vi "Vision Auto Target_Old.vi"(11 "navX Device":T1={"Interface"={"Protocol"=enum."SERIAL", "Update Rate (4Hz-60Hz)"=4, "navX Open TypeDef"=variant}, "Notify Packet"=refnum, "Loop VI Refnum"=refnum, "Ready to Close Occurrence Refnum"=refnum} {"Interface"."Update Rate (4Hz-60Hz)" min=4 max=60 step=1}) -> ()   [LabVIEW 2015]
uses:
  NavX/navX Library v2/TypeDefs/Z900_navX_DeviceTypeDef.ctl
  NavX/navX Library v2/TypeDefs/Z900_navX_ProtocolTypeDef.ctl
  NavX/navX Library v2/TypeDefs/Z900_navX_NotifyPacketTypeDef.ctl
  NavX/navX Library v2/TypeDefs/Z900_navX_ActionTypeDef.ctl
  Team Code/Robot Global Data.vi
  <vilib>/Rock Robotics/Network Tables/NT Write Number.vi
  NavX/navX Library v2/navX Library v2.lvlib
panel:
  in  "Y Gain":dbl=6.5
  in  "Y at Defenses":dbl=-0.4
  in  "InvGain":dbl=80.0
  in  "minimumVisionValue":dbl=0.45
  out "Waveform Chart":cluster{"VisionGyroTarget":dbl, dbl, dbl}(graph)
  out "VisionState":enum16{"Disabled", "Enable", "Suspended", "PID"}(ring)
  in  "Offset":dbl=0.05
  # "0.05 = 4 inches from defenses\n- = Left\n+ = Right"
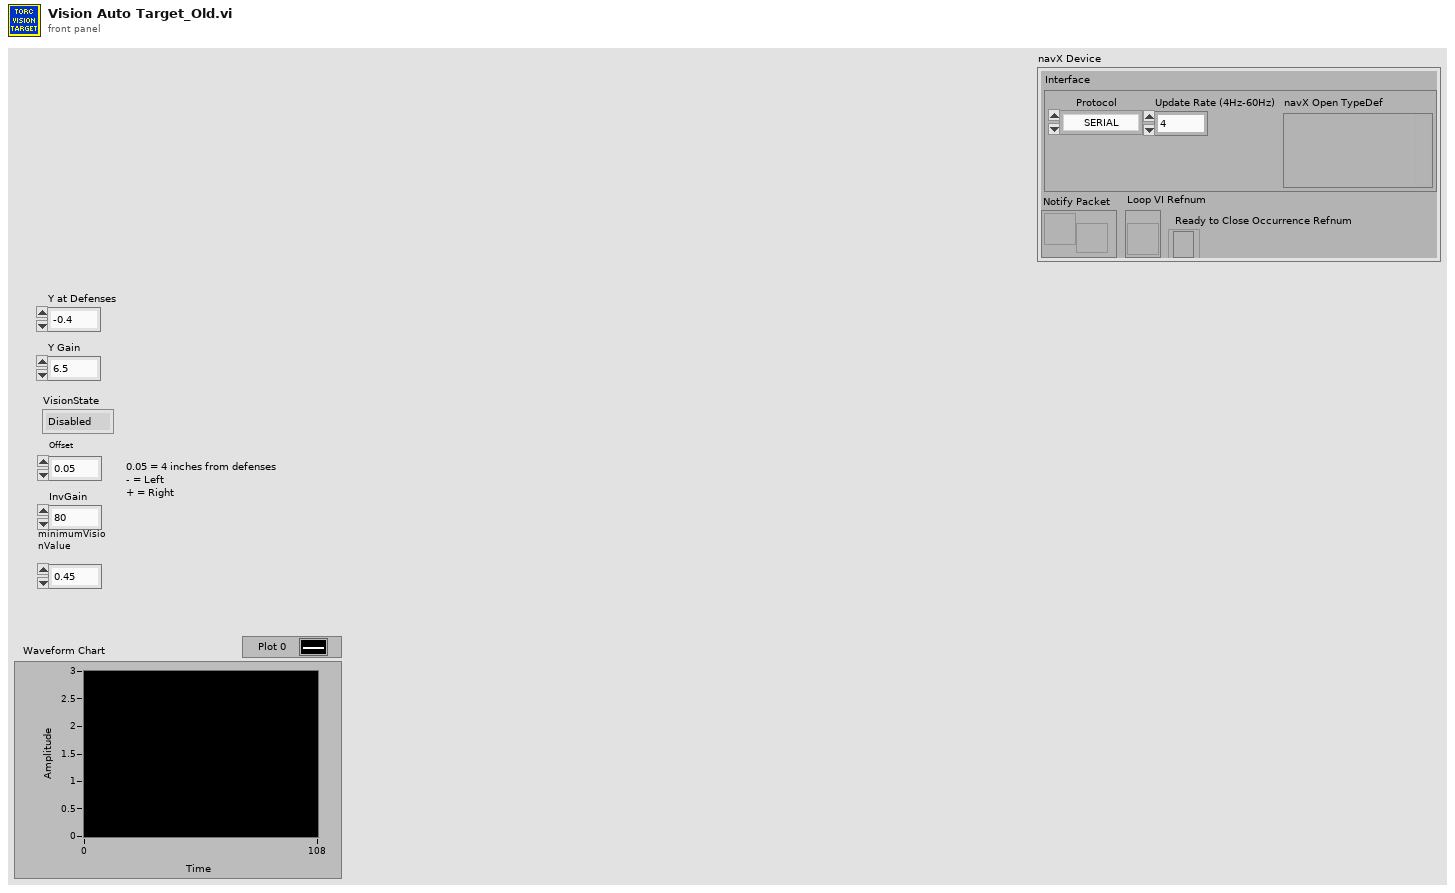
[diagram p1: front panel]
types:
  T1 = typedef "navX Library v2.lvlib/Z900_navX_DeviceTypeDef.ctl" = cluster{"Interface":cluster{"Protocol":T2, "Update Rate (4Hz-60Hz)":u8, "navX Open TypeDef":variant}, "Notify Packet":refnum<notifier>, "Loop VI Refnum":refnum<vi>, "Ready to Close Occurrence Refnum":refnum<k4>}
  T2 = typedef "navX Library v2.lvlib/Z900_navX_ProtocolTypeDef.ctl" = enum16{"SERIAL", "I2C", "SPI"}
  T3 = cluster{"Yaw":dbl, "Roll":dbl, "Pitch":dbl, "Heading":dbl, "Fused Heading":dbl}
  T4 = cluster{"Distance (ft)":dbl, "Center":cluster{dbl, dbl}, "Normalized Rect":cluster{"Numeric":dbl, "Numeric 2":dbl, "Numeric 3":dbl, "Numeric 5":dbl}}[]
  T5 = cluster{"Detected Targets[0]":cluster{"Distance (ft)":dbl, "Center":cluster{dbl, dbl}, "Normalized Rect":cluster{"Numeric":dbl, "Numeric 2":dbl, "Numeric 3":dbl, "Numeric 5":dbl}}, "Detected Targets[1]":cluster{"Distance (ft)":dbl, "Center":cluster{dbl, dbl}, "Normalized Rect":cluster{"Numeric":dbl, "Numeric 2":dbl, "Numeric 3":dbl, "Numeric 5":dbl}}, "Detected Targets[2]":cluster{"Distance (ft)":dbl, "Center":cluster{dbl, dbl}, "Normalized Rect":cluster{"Numeric":dbl, "Numeric 2":dbl, "Numeric 3":dbl, "Numeric 5":dbl}}, "Detected Targets[3]":cluster{"Distance (ft)":dbl, "Center":cluster{dbl, dbl}, "Normalized Rect":cluster{"Numeric":dbl, "Numeric 2":dbl, "Numeric 3":dbl, "Numeric 5":dbl}}, "Detected Targets[4]":cluster{"Distance (ft)":dbl, "Center":cluster{dbl, dbl}, "Normalized Rect":cluster{"Numeric":dbl, "Numeric 2":dbl, "Numeric 3":dbl, "Numeric 5":dbl}}, "Detected Targets[5]":cluster{"Distance (ft)":dbl, "Center":cluster{dbl, dbl}, "Normalized Rect":cluster{"Numeric":dbl, "Numeric 2":dbl, "Numeric 3":dbl, "Numeric 5":dbl}}, "Detected Targets[6]":cluster{"Distance (ft)":dbl, "Center":cluster{dbl, dbl}, "Normalized Rect":cluster{"Numeric":dbl, "Numeric 2":dbl, "Numeric 3":dbl, "Numeric 5":dbl}}, "Detected Targets[7]":cluster{"Distance (ft)":dbl, "Center":cluster{dbl, dbl}, "Normalized Rect":cluster{"Numeric":dbl, "Numeric 2":dbl, "Numeric 3":dbl, "Numeric 5":dbl}}, "Detected Targets[8]":cluster{"Distance (ft)":dbl, "Center":cluster{dbl, dbl}, "Normalized Rect":cluster{"Numeric":dbl, "Numeric 2":dbl, "Numeric 3":dbl, "Numeric 5":dbl}}}
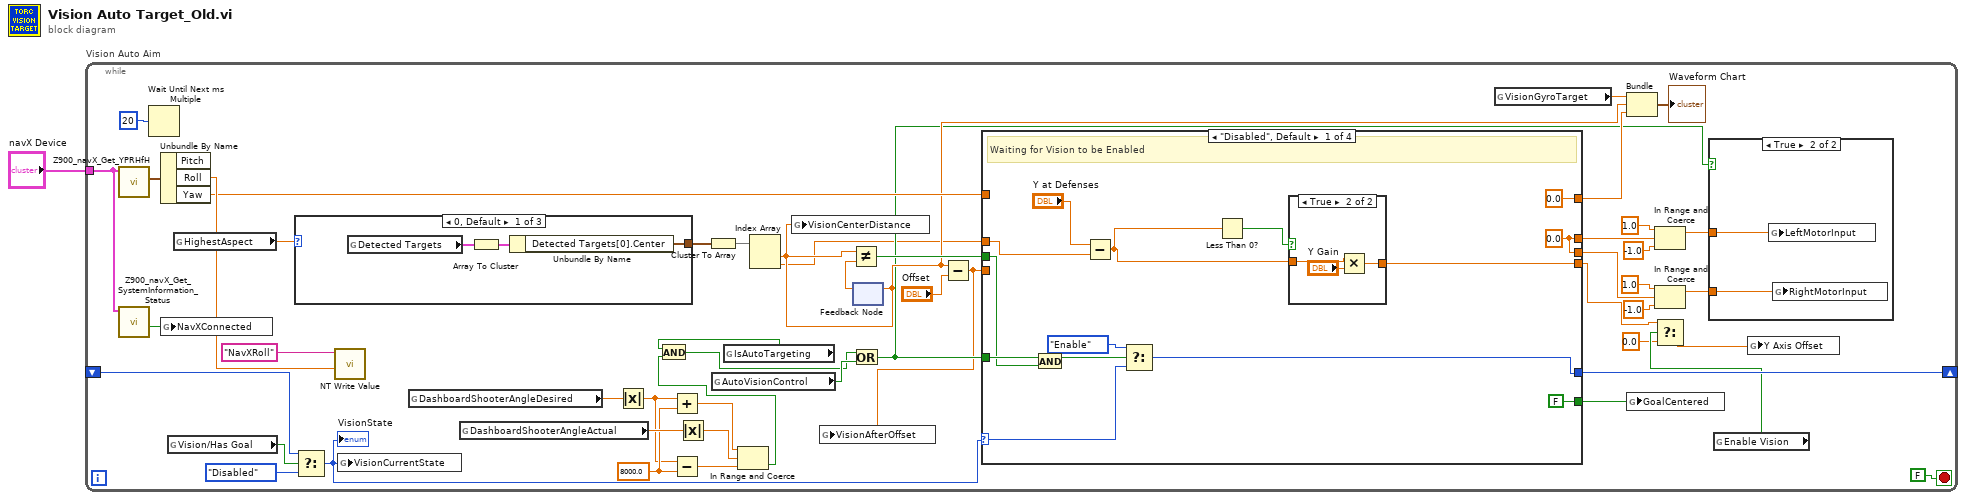
[diagram p0: block diagram]
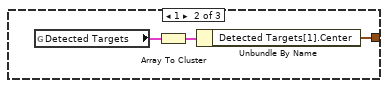
[diagram p2: hidden frame]
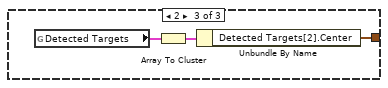
[diagram p3: hidden frame]
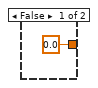
[diagram p5: hidden frame]
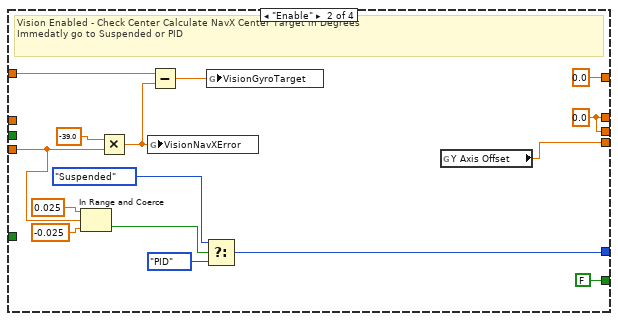
[diagram p6: hidden frame]
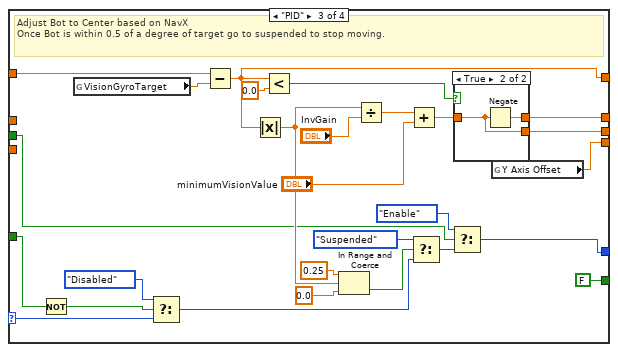
[diagram p7: hidden frame]
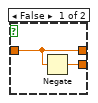
[diagram p8: hidden frame]
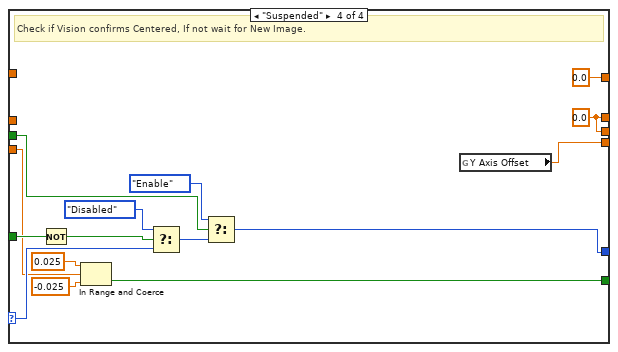
[diagram p9: hidden frame]
diagram:
  n1 = while "Vision Auto Aim" {
    tunnel: "navX Device" -> [w45]
    shift-right: [w48] -> _
    shift-left: _ -> [w26]
    stop <- FALSE stop-if-true
    w12 = 8000.0 ("y")
    n2 = call "Z900_navX_Get_YPRHfH.vi"("navX Device"=w45) -> ("YRPHfH"=w49:T3)  [unwired: 7 in, 3 out]
    n3 = call "Z900_navX_Get_SystemInformation_Status.vi"("navX Device"=w45) -> ("Connected"=w28:bool)  [unwired: 7 in, 3 out]
    n4 = Wait Until Next ms Multiple(millisecond multiple=u32 20 ("milliseconds to wait")) -> ()  [unwired: 1 out]
    n5 = Unbundle By Name(w49) -> ("Roll"=w47:dbl, "Yaw"=w21:dbl)  [unwired: 1 out]
    n6 = global write "Robot Global Data.vi" "NavXConnected"(w28) -> ()
    n7 = global read "Robot Global Data.vi" "Vision/Has Goal"() -> (w25:bool)
    n8 = global read "Robot Global Data.vi" "HighestAspect"() -> (w23:dbl)
    n9 = case shown="0, Default" w23 {
      tunnel: [w52 w55 w58] -> w32
      frame 0, Default {
        n10 = global read "Robot Global Data.vi" "Detected Targets"() -> (w53:T4)
        n11 = Array To Cluster(array=w53) -> (cluster=w54:T5)
        n12 = Unbundle By Name(w54) -> ("Detected Targets[0].Center"=w52:cluster{dbl, dbl})
      }
      frame 1 {
        n13 = global read "Robot Global Data.vi" "Detected Targets"() -> (w56:T4)
        n14 = Array To Cluster(array=w56) -> (cluster=w57:T5)
        n15 = Unbundle By Name(w57) -> ("Detected Targets[1].Center"=w55:cluster{dbl, dbl})
      }
      frame 2 {
        n16 = global read "Robot Global Data.vi" "Detected Targets"() -> (w59:T4)
        n17 = Array To Cluster(array=w59) -> (cluster=w60:T5)
        n18 = Unbundle By Name(w60) -> ("Detected Targets[2].Center"=w58:cluster{dbl, dbl})
      }
    }
    n19 = Select(t=w26, s=w25, f=enum16{"Disabled", "Enable", "Suspended", "PID"}."Disabled" ("t")) -> (s? t:f=w27:enum16{"Disabled", "Enable", "Suspended", "PID"})
    "VisionState" <- w27
    n20 = call-poly <vilib>:"NT Write Value.vi"("Numeric"=w47, "Name"="NavXRoll") -> ()  [unwired: 9 in, 1 out]
    n21 = global write "Robot Global Data.vi" "VisionCurrentState"(w27) -> ()
    n22 = global read "Robot Global Data.vi" "DashboardShooterAngleDesired"() -> (w14:dbl)
    n23 = global read "Robot Global Data.vi" "DashboardShooterAngleActual"() -> (w17:dbl)
    n24 = Absolute Value(x=w14) -> (abs(x)=w11:dbl)
    n25 = Add(x=w11, y=w12) -> (x+y=w16:dbl)
    n26 = Subtract(x=w11, y=w12) -> (x-y=w15:dbl)
    n27 = Absolute Value(x=w17) -> (abs(x)=w13:dbl)
    n28 = Cluster To Array(cluster=w32) -> (array=w44:dbl[])
    n29 = global read "Robot Global Data.vi" "AutoVisionControl"() -> (w29:bool)
    n30 = global read "Robot Global Data.vi" "IsAutoTargeting"() -> (w10:bool)
    n31 = In Range and Coerce(upper limit=w16, x=w13, lower limit=w15) -> (In Range?=w9:bool)  [unwired: 1 out]
    n32 = And(x=w10, y=w9) -> (x .and. y?=w8:bool)
    n33 = Index Array(array=w44) -> (element #1=w20:dbl, element #2=w6:dbl)  [unwired: 2 in]
    n34 = global write "Robot Global Data.vi" "VisionCenterDistance"(w20) -> ()
    n35 = Or(x=w8, y=w29) -> (x .or. y?=w18:bool)
    n36 = feedback-in #1(w20) -> ()
    n37 = feedback #1() -> (w30:dbl)  [unwired: 1 in]
    n38 = Not Equal?(x=w20, y=w30) -> (x != y?=w31:bool)
    n39 = Subtract(x=w20, y="Offset") -> (x-y=w7:dbl)
    n40 = global write "Robot Global Data.vi" "VisionAfterOffset"(w7) -> ()
    n41 = case shown="\"Disabled\", Default" w27 {
      selector: w27 -> [w76 _ w99 w131]
      tunnel: w18 -> [w72 _ w102 w133]
      tunnel: [w74 w93 w104 w132] -> w48
      tunnel: w21 -> [_ w86 w111 _]
      tunnel: [FALSE FALSE FALSE w129] -> w19
      tunnel: w7 -> [_ w82 _ w128]
      tunnel: [w71 w89 w113 w141] -> w39
      tunnel: [w71 w89 w114 w141] -> w43
      tunnel: [0.0 0.0 w110 0.0] -> w34
      tunnel: w31 -> [w68 _ w98 w130]
      tunnel: w6 -> [w64 _ _ _]
      tunnel: [w65 w81 w97 w127] -> w4
      frame "Disabled", Default {
        w71 = 0.0
        # "Waiting for Vision to be Enabled"
        n42 = And(x=w72, y=w68) -> (x .and. y?=w69:bool)
        n43 = Subtract(x="Y at Defenses", y=w64) -> (x-y=w66:dbl)
        n44 = Select(t=enum16{"Disabled", "Enable", "Suspended", "PID"}."Enable", s=w69, f=w76) -> (s? t:f=w74:enum16{"Disabled", "Enable", "Suspended", "PID"})
        n45 = Less Than 0?(x=w66) -> (x < 0?=w67:bool)
        n46 = case shown="True" w67 {
          tunnel: w66 -> [_ w79]
          tunnel: [0.0 w78] -> w65
          frame False {
          }
          frame True {
            n47 = Multiply(x=w79, y="Y Gain") -> (x*y=w78:dbl)
          }
        }
      }
      frame "Enable" {
        w89 = 0.0 ("LeftMotorOutput")
        # "Vision Enabled - Check Center Calculate NavX Center Target in Degrees\nImmedatly go to Suspended or PID"
        n48 = In Range and Coerce(upper limit=0.025, x=w82, lower limit=-0.025) -> (In Range?=w84:bool)  [unwired: 1 out]
        n49 = Multiply(x=-39.0, y=w82) -> (x*y=w85:dbl)
        n50 = global write "Robot Global Data.vi" "VisionNavXError"(w85) -> ()
        n51 = Subtract(x=w86, y=w85) -> (x-y=w88:dbl)
        n52 = Select(t=enum16{"Disabled", "Enable", "Suspended", "PID"}."Suspended", s=w84, f=enum16{"Disabled", "Enable", "Suspended", "PID"}."PID" ("t")) -> (s? t:f=w93:enum16{"Disabled", "Enable", "Suspended", "PID"})
        n53 = global write "Robot Global Data.vi" "VisionGyroTarget"(w88) -> ()
        n54 = global read "Robot Global Data.vi" "Y Axis Offset"() -> (w81:dbl)
      }
      frame "PID" {
        # "Adjust Bot to Center based on NavX\nOnce Bot is within 0.5 of a degree of target go to suspended to stop moving."
        n55 = Not(x=w102) -> (.not. x?=w101:bool)
        n56 = global read "Robot Global Data.vi" "VisionGyroTarget"() -> (w120:dbl)
        n57 = Select(t=enum16{"Disabled", "Enable", "Suspended", "PID"}."Disabled", s=w101, f=w99) -> (s? t:f=w100:enum16{"Disabled", "Enable", "Suspended", "PID"})
        n58 = Subtract(x=w111, y=w120) -> (x-y=w110:dbl)
        n59 = Absolute Value(x=w110) -> (abs(x)=w108:dbl)
        n60 = Less?(x=w110, y=0.0) -> (x < y?=w116:bool)
        n61 = In Range and Coerce(upper limit=0.25, x=w108, lower limit=0.0) -> (In Range?=w96:bool)  [unwired: 1 out]
        n62 = Divide(x=w108, y="InvGain") -> (x/y=w118:dbl)
        n63 = Add(x=w118, y="minimumVisionValue") -> (x+y=w115:dbl)
        n64 = Select(t=enum16{"Disabled", "Enable", "Suspended", "PID"}."Suspended", s=w96, f=w100) -> (s? t:f=w105:enum16{"Disabled", "Enable", "Suspended", "PID"})
        n65 = Select(t=enum16{"Disabled", "Enable", "Suspended", "PID"}."Enable", s=w98, f=w105) -> (s? t:f=w104:enum16{"Disabled", "Enable", "Suspended", "PID"})
        n66 = case shown="True" w116 {
          tunnel: w115 -> [w124 w125]
          tunnel: [w123 w125] -> w114
          tunnel: [w124 w126] -> w113
          frame False {
            n67 = Negate(x=w124) -> (-x=w123:dbl)
          }
          frame True {
            n68 = Negate(x=w125) -> (-x=w126:dbl)
          }
        }
        n69 = global read "Robot Global Data.vi" "Y Axis Offset"() -> (w97:dbl)
      }
      frame "Suspended" {
        w141 = 0.0 ("LeftMotorOutput")
        # "Check if Vision confirms Centered, If not wait for New Image."
        n70 = Not(x=w133) -> (.not. x?=w134:bool)
        n71 = In Range and Coerce(upper limit=0.025, x=w128, lower limit=-0.025) -> (In Range?=w129:bool)  [unwired: 1 out]
        n72 = Select(t=enum16{"Disabled", "Enable", "Suspended", "PID"}."Disabled" ("f"), s=w134, f=w131) -> (s? t:f=w136:enum16{"Disabled", "Enable", "Suspended", "PID"})
        n73 = Select(t=enum16{"Disabled", "Enable", "Suspended", "PID"}."Enable" ("f"), s=w130, f=w136) -> (s? t:f=w132:enum16{"Disabled", "Enable", "Suspended", "PID"})
        n74 = global read "Robot Global Data.vi" "Y Axis Offset"() -> (w127:dbl)
      }
    }
    n75 = global read "Robot Global Data.vi" "VisionGyroTarget"() -> (w35:dbl)
    n76 = Bundle("VisionGyroTarget"=w35, w20, w34) -> (→"Waveform Chart":cluster{"VisionGyroTarget":dbl, dbl, dbl})  [unwired: 1 in]
    n77 = global write "Robot Global Data.vi" "GoalCentered"(w19) -> ()
    n78 = In Range and Coerce(upper limit=1.0, x=w39, lower limit=-1.0) -> (coerced(x)=w37:dbl)  [unwired: 1 out]
    n79 = In Range and Coerce(upper limit=1.0, x=w43, lower limit=-1.0) -> (coerced(x)=w36:dbl)  [unwired: 1 out]
    n80 = case shown="True" w18 {
      tunnel: w36 -> [_ w61]
      tunnel: w37 -> [_ w62]
      frame False {
      }
      frame True {
        n81 = global write "Robot Global Data.vi" "LeftMotorInput"(w62) -> ()
        n82 = global write "Robot Global Data.vi" "RightMotorInput"(w61) -> ()
      }
    }
    n83 = global read "Robot Global Data.vi" "Enable Vision"() -> (w3:bool)
    n84 = Select(t=w4, s=w3, f=0.0) -> (s? t:f=w5:dbl)
    n85 = global write "Robot Global Data.vi" "Y Axis Offset"(w5) -> ()
  }
